vi "TCP Write.vi"(8 "error in":errorcluster, 9 "timeout":i32, 10 "data":u8[](array[numeric]), 11 "connection ID":refnum<k5>) -> (0 "error out":errorcluster, 1 "timed out?":bool)   [LabVIEW 2013, in "Modbus Library - Advance.lvlib" / "TCP Shared Components.lvlib"]
doc: "This VI writes a set of data to a TCP connection and checks for errors. It is a wrapper for standard functionality."
uses:
  TCP Shared Components.lvlib
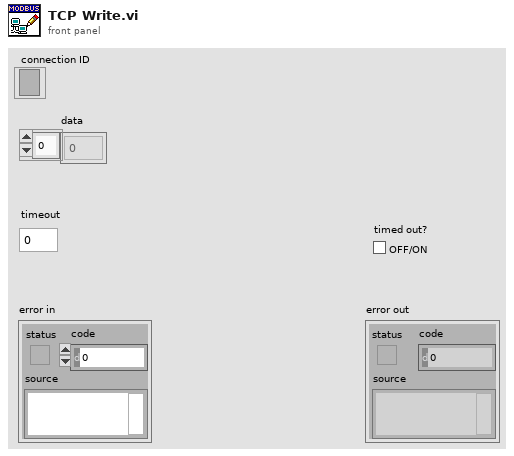
[diagram p1: front panel]
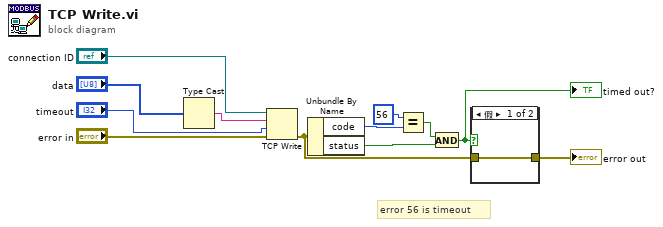
[diagram p0: block diagram]
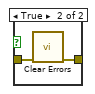
[diagram p2: hidden frame]
diagram:
  # "error 56 is timeout"
  n1 = Type Cast(x="data") -> (*(type *) &x=w6:string)  [unwired: 1 in]
  n2 = TCP Write(connection ID="connection ID", data in=w6, error in (no error)="error in", 9:"timeout") -> (error out=w1:errorcluster)  [unwired: 2 out]
  n3 = Unbundle By Name(w1) -> ("code"=w4:i32, "status"=w2:bool)
  n4 = Equal?(x=56, y=w4) -> (x = y?=w5:bool)
  n5 = And(x=w5, y=w2) -> (x .and. y?=w8:bool)
  "timed out?" <- w8
  n6 = case shown="假" w8 {
    tunnel: w1 -> [w13 w15]
    tunnel: [w13 w14] -> w11
    frame False {
    }
    frame True {
      n7 = call <vilib>:"Clear Errors.vi"("error in (no error)"=w15) -> ("error out"=w14:errorcluster)  [unwired: 6 in]
    }
  }
  "error out" <- w11
